vi "GA Get Capture Mode.vi"(8 "error in (no error)":errorcluster caption="错误输入（无错误）", 9 "nCount":i16, 10 "pMode":i16, 11 "nEncodeNum":i16) -> (0 "error out":errorcluster caption="错误输出", 2 "pMode out":i16, 3 "function return":i32)   [LabVIEW 2015, in "GAS.lvlib"]
doc: "extern \"C\" __declspec(dllimport) int GA_GetCaptureMode(short nEncodeNum,short *pMode,short nCount=1);"
uses:
  <userlib>/BP_GAS/GAS.lvlib
  <userlib>/BP_GAS/GAS.dll
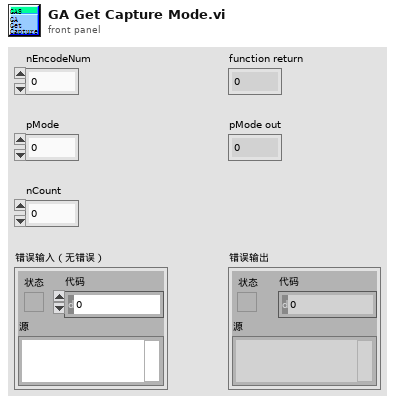
[diagram p1: front panel]
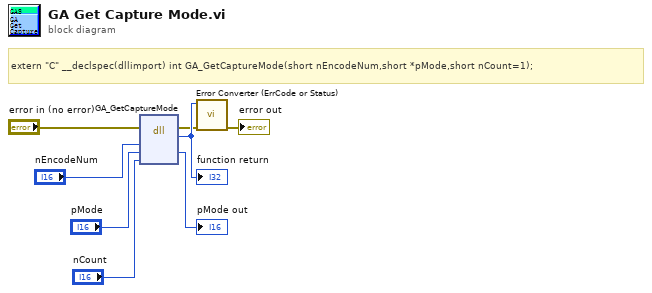
[diagram p0: block diagram]
diagram:
  # "extern \"C\" __declspec(dllimport) int GA_GetCaptureMode(short nEncodeNum,short *pMode,short nCount=1);"
  n1 = dll-call lib="E:/Program Files (x86)/National Instruments/LabVIEW 2015/user.lib/BP_GAS/GAS.*" fn="GA_GetCaptureMode"(error in="error in (no error)", "nEncodeNum"="nEncodeNum", "pMode"="pMode", "nCount"="nCount") -> (error out=w2:errorcluster, w8:i32, "pMode"=→"pMode out":i16)  [unwired: 4 in, 1 out]
  "function return" <- w8
  n2 = call "Error Converter (ErrCode or Status).vi"("error in (no error)"=w2, "error code"=w8) -> ("error out"=→"error out":errorcluster)  [unwired: 9 in]
